vi "Set Wheel Separation.vi"(6 "subpanel to main command event":T1, 8 "error in (no error)":errorcluster, 9 "wheel separation length":dbl, 10 "wheel separation width":dbl, 11 "steering frame ref in":refnum<data-value>) -> (0 "error out":errorcluster, 3 "steering frame ref out":refnum<data-value>)   [LabVIEW 2017, in "NI_Robotics_Configure Steering Frame.lvlib" / "Ackermann Frame Subpanel.lvlib"]
uses:
  <vilib>/robotics/Dialog/Configure Steering Frame/Ackermann Frame Subpanel/Ackermann Frame Subpanel.lvlib
  <vilib>/robotics/Steering/Ackermann Steering Frame/NI_Robotics_Ackermann Steering Frame.lvclass
  c:/Program Files (x86)/National Instruments/LabVIEW 2017/vi.lib/robotics/Steering/Steering Frame/NI_Robotics_Steering Frame.lvclass
  <vilib>/robotics/Dialog/Configure Steering Frame/Subpanel to Main Command Event.ctl
  <vilib>/robotics/Dialog/Configure Steering Frame/Subpanel to Main Command.ctl
  <vilib>/robotics/Steering/Steering Frame/NI_Robotics_Steering Frame.lvclass/NI_Robotics_Steering Frame.ctl
  <vilib>/robotics/Steering/Wheel/NI_Robotics_Wheel.lvclass/NI_Robotics_Wheel.ctl
  <vilib>/robotics/Steering/Ackermann Steering Frame/NI_Robotics_Ackermann Steering Frame.lvclass/NI_Robotics_Ackermann Steering Frame.ctl
  <vilib>/robotics/Steering/Ackermann Steering Frame/Wheel Separation to Frame Positions.vi
  <vilib>/robotics/Steering/Steering Frame/Reposition Wheels.vi
  <vilib>/robotics/Dialog/Configure Steering Frame/Generate Subpanel to Main Event.vi
  <vilib>/robotics/Steering/Wheel/Update Steering to Wheel Frame Transform.vi
  <vilib>/Analysis/coordinate.llb/Wrap Angle.vi
  <vilib>/Analysis/coordinate.llb/Wrap Angle (scalar).vi
  <vilib>/robotics/Dialog/Configure Steering Frame/NI_Robotics_Configure Steering Frame.lvlib
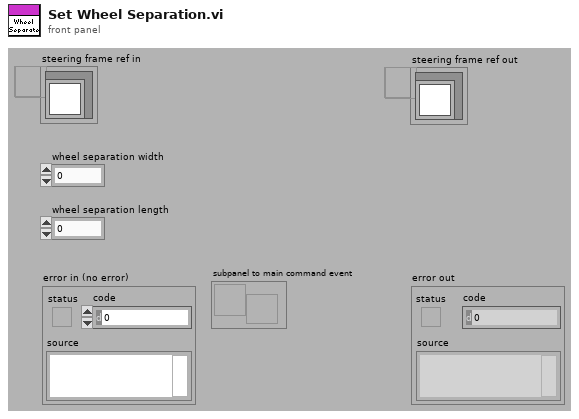
[diagram p1: front panel]
types:
  T1 = typedef "NI_Robotics_Configure Steering Frame.lvlib/Subpanel to Main Command Event.ctl" = refnum<user-event>
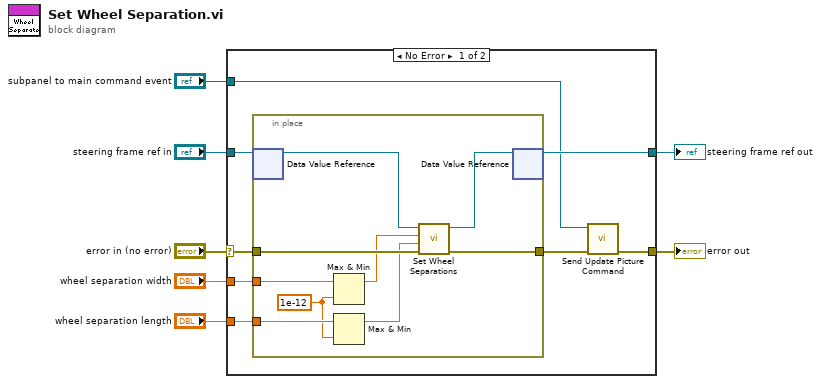
[diagram p0: block diagram]
diagram:
  n1 = case shown="No Error" "error in (no error)" {
    selector: "error in (no error)" -> [w14 w25]
    tunnel: "steering frame ref in" -> [w15 w26]
    tunnel: [w12 w26] -> w5
    tunnel: [w8 w25] -> w4
    tunnel: "subpanel to main command event" -> [w10 _]
    tunnel: "wheel separation width" -> [w13 _]
    tunnel: "wheel separation length" -> [w11 _]
    frame No Error {
      n2 = in-place {
        in-place-border: w14 -> [w24]
        in-place-border: w13 -> [w20]
        in-place-border: [w23] -> w9
        in-place-border: w11 -> [w19]
        w18 = 1e-12 ("y")
        n3 = in-place-dvr #1(w15) -> (w21:refnum<class "NI_Robotics_Ackermann Steering Frame.lvclass">)  [unwired: 1 out]
        n4 = Max & Min(x=w20, y=w18) -> (max(x,y)=w17:dbl)  [unwired: 1 out]
        n5 = Max & Min(x=w19, y=w18) -> (max(x,y)=w16:dbl)  [unwired: 1 out]
        n6 = call <vilib>:"Set Wheel Separations.vi"("error in (no error)"=w24, "wheel separation length"=w16, "wheel separation width"=w17, "ackermann steering frame in"=w21) -> ("error out"=w23:errorcluster, "ackermann steering frame out"=w22:refnum<class "NI_Robotics_Ackermann Steering Frame.lvclass">)  [unwired: 6 in]
        n7 = in-place-dvr #1(w22) -> (w12:refnum<data-value>)  [unwired: 1 out]
      }
      n8 = call <vilib>:"Send Update Picture Command.vi"("error in (no error)"=w9, "subpanel to main command event"=w10) -> ("error out"=w8:errorcluster)  [unwired: 9 in]
    }
    frame Error {
    }
  }
  "steering frame ref out" <- w5
  "error out" <- w4
